vi "Configure Trigger Holdoff.vi"(7 "Holdoff Mode (0: Fixed)":i32(ring) items=["Fixed", "Random"], 8 "error in (no error)":errorcluster, 9 "Holdoff Max (10.0 s)":dbl=10.0, 10 "Holdoff Min (1E-7 s)":dbl=1e-07, 11 "VISA resource name":refnum<visa-resource-name>) -> (0 "error out":errorcluster, 3 "VISA resource name out":refnum<visa-resource-name>)   [LabVIEW 2020, in "Agilent 90000 Series.lvlib"]
doc: "Configures the holdoff of triggers."
uses:
  Agilent 90000 Series.lvlib
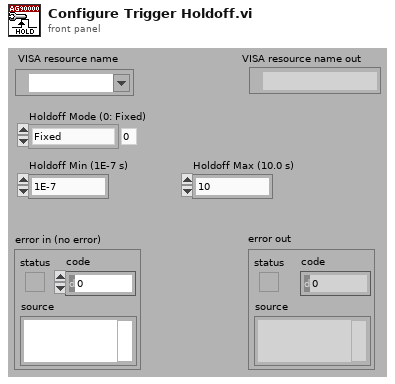
[diagram p1: front panel]
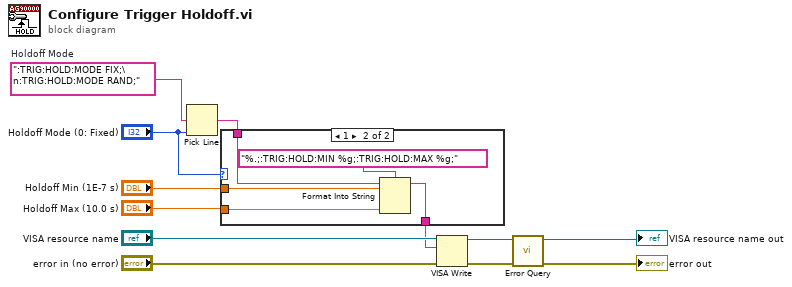
[diagram p0: block diagram]
diagram:
  w12 = ":TRIG:HOLD:MODE FIX;\n:TRIG:HOLD:MODE RAND;"  # Holdoff Mode
  n1 = Pick Line(multi-line string=w12, line index="Holdoff Mode (0: Fixed)") -> (output string=w3:string)  [unwired: 1 out]
  n2 = case shown="1" "Holdoff Mode (0: Fixed)" {
    tunnel: [w13 w18] -> w5
    tunnel: "Holdoff Min (1E-7 s)" -> [_ w16]
    tunnel: w3 -> [w13 w15]
    tunnel: "Holdoff Max (10.0 s)" -> [_ w14]
    frame 0, Default {
    }
    frame 1 {
      n3 = Format Into String(format string="%.;:TRIG:HOLD:MIN %g;:TRIG:HOLD:MAX %g;", initial string=w15, w16, w14) -> (resulting string=w18:string)  [unwired: 1 in, 1 out]
    }
  }
  n4 = VISA Write(VISA resource name="VISA resource name", write buffer=w5, error in (no error)="error in (no error)") -> (VISA resource name out=w9:refnum<visa-resource-name>, error out=w8:errorcluster)  [unwired: 1 out]
  n5 = call "Error Query.vi"("error in (no error)"=w8, "VISA resource name"=w9) -> ("error out"=→"error out":errorcluster, "VISA resource name out"=→"VISA resource name out":refnum<visa-resource-name>)  [unwired: 8 out]
